vi "saveSpinInfo.vi"(6 "error in (no error)":errorcluster, 7 "folder":path, 8 "direction":bool, 9 "increment":sgl, 10 "angleToMove":sgl, 11 "startAngle":sgl) -> (4 "error out":errorcluster)   [LabVIEW 2014]
panel:
  # "CW"
  # "CCW"
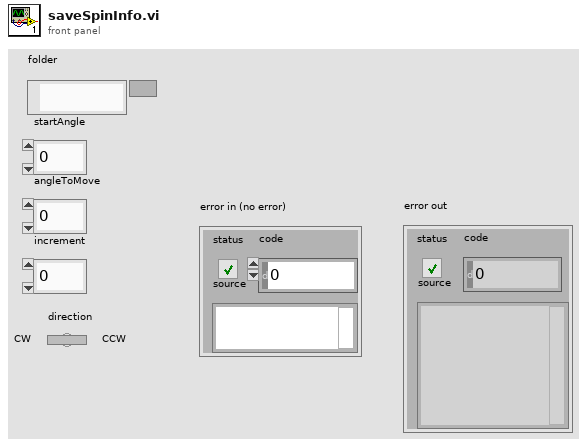
[diagram p1: front panel]
types:
  T1 = enum16{"open", "replace", "create", "open or create", "replace or create", "replace or create with confirmation"}
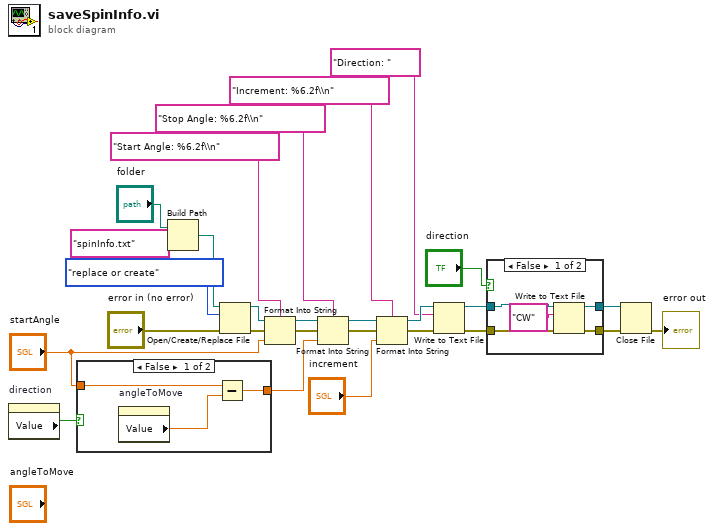
[diagram p0: block diagram]
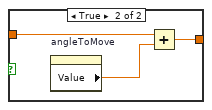
[diagram p2: hidden frame]
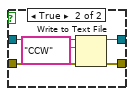
[diagram p3: hidden frame]
diagram:
  n1 = property on="direction" class="Bool (strict)"() -> ("Value"=w3:bool)  [unwired: 2 in, 2 out]
  n2 = case shown="False" w3 {
    tunnel: "startAngle" -> [w29 w32]
    tunnel: [w28 w31] -> w1
    frame False {
      n3 = property on="angleToMove" class="DigNum (strict)"() -> ("Value"=w30:sgl)  [unwired: 2 in, 2 out]
      n4 = Subtract(x=w29, y=w30) -> (x-y=w28:sgl)
    }
    frame True {
      n5 = property on="angleToMove" class="DigNum (strict)"() -> ("Value"=w33:sgl)  [unwired: 2 in, 2 out]
      n6 = Add(x=w32, y=w33) -> (x+y=w31:sgl)
    }
  }
  n7 = Build Path(base path="folder", name or relative path="spinInfo.txt") -> (appended path=w25:path)
  n8 = Open/Create/Replace File(file path (use dialog)=w25, error in="error in (no error)", operation (0:open)=T1."replace or create") -> (refnum out=w23:refnum<file>, error out=w21:errorcluster)  [unwired: 3 in, 1 out]
  n9 = Format Into String(format string="Start Angle: %6.2f\\n", initial string=w23, error in=w21, "startAngle") -> (resulting string=w18:refnum<file>, error out=w19:errorcluster)
  n10 = Format Into String(format string="Stop Angle: %6.2f\\n", initial string=w18, error in=w19, w1) -> (resulting string=w16:refnum<file>, error out=w15:errorcluster)
  n11 = Format Into String(format string="Increment: %6.2f\\n", initial string=w16, error in=w15, "increment") -> (resulting string=w13:refnum<file>, error out=w8:errorcluster)
  n12 = Write to Text File(file (use dialog)=w13, text="Direction: " ("format string"), error in=w8) -> (refnum out=w12:refnum<file>, error out=w6:errorcluster)  [unwired: 1 in, 1 out]
  n13 = case shown="False" "direction" {
    tunnel: w12 -> [w37 w43]
    tunnel: w6 -> [w36 w41]
    tunnel: [w38 w42] -> w11
    tunnel: [w34 w39] -> w10
    frame False {
      n14 = Write to Text File(file (use dialog)=w37, text="CW" ("format string"), error in=w36) -> (refnum out=w38:refnum<file>, error out=w34:errorcluster)  [unwired: 1 in, 1 out]
    }
    frame True {
      n15 = Write to Text File(file (use dialog)=w43, text="CCW" ("format string"), error in=w41) -> (refnum out=w42:refnum<file>, error out=w39:errorcluster)  [unwired: 1 in, 1 out]
    }
  }
  n16 = Close File(refnum=w11, error in=w10) -> (error out=→"error out":errorcluster)  [unwired: 1 out]
